vi "ZStepperPositionTest.vi"() -> ()   [LabVIEW 2014]
uses:
  inc/ThorZStepper.lvlib
panel:
  out "ZPosSlider":dbl(slide) caption="Z (mm)" min=-2.0 max=16.0 scale=-2.0..2.0
  in  "Z Stop":bool
  in  "Z Set Zero":bool
  in  "Tear Down Device and Stop Communication":bool
  out "status":i32
  in  "Move to New ZPos":bool
  in  "New ZPos (um)":dbl
  out "Current ZPos (mm)":dbl
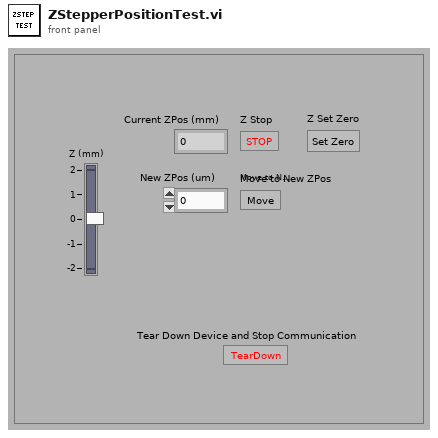
[diagram p1: front panel]
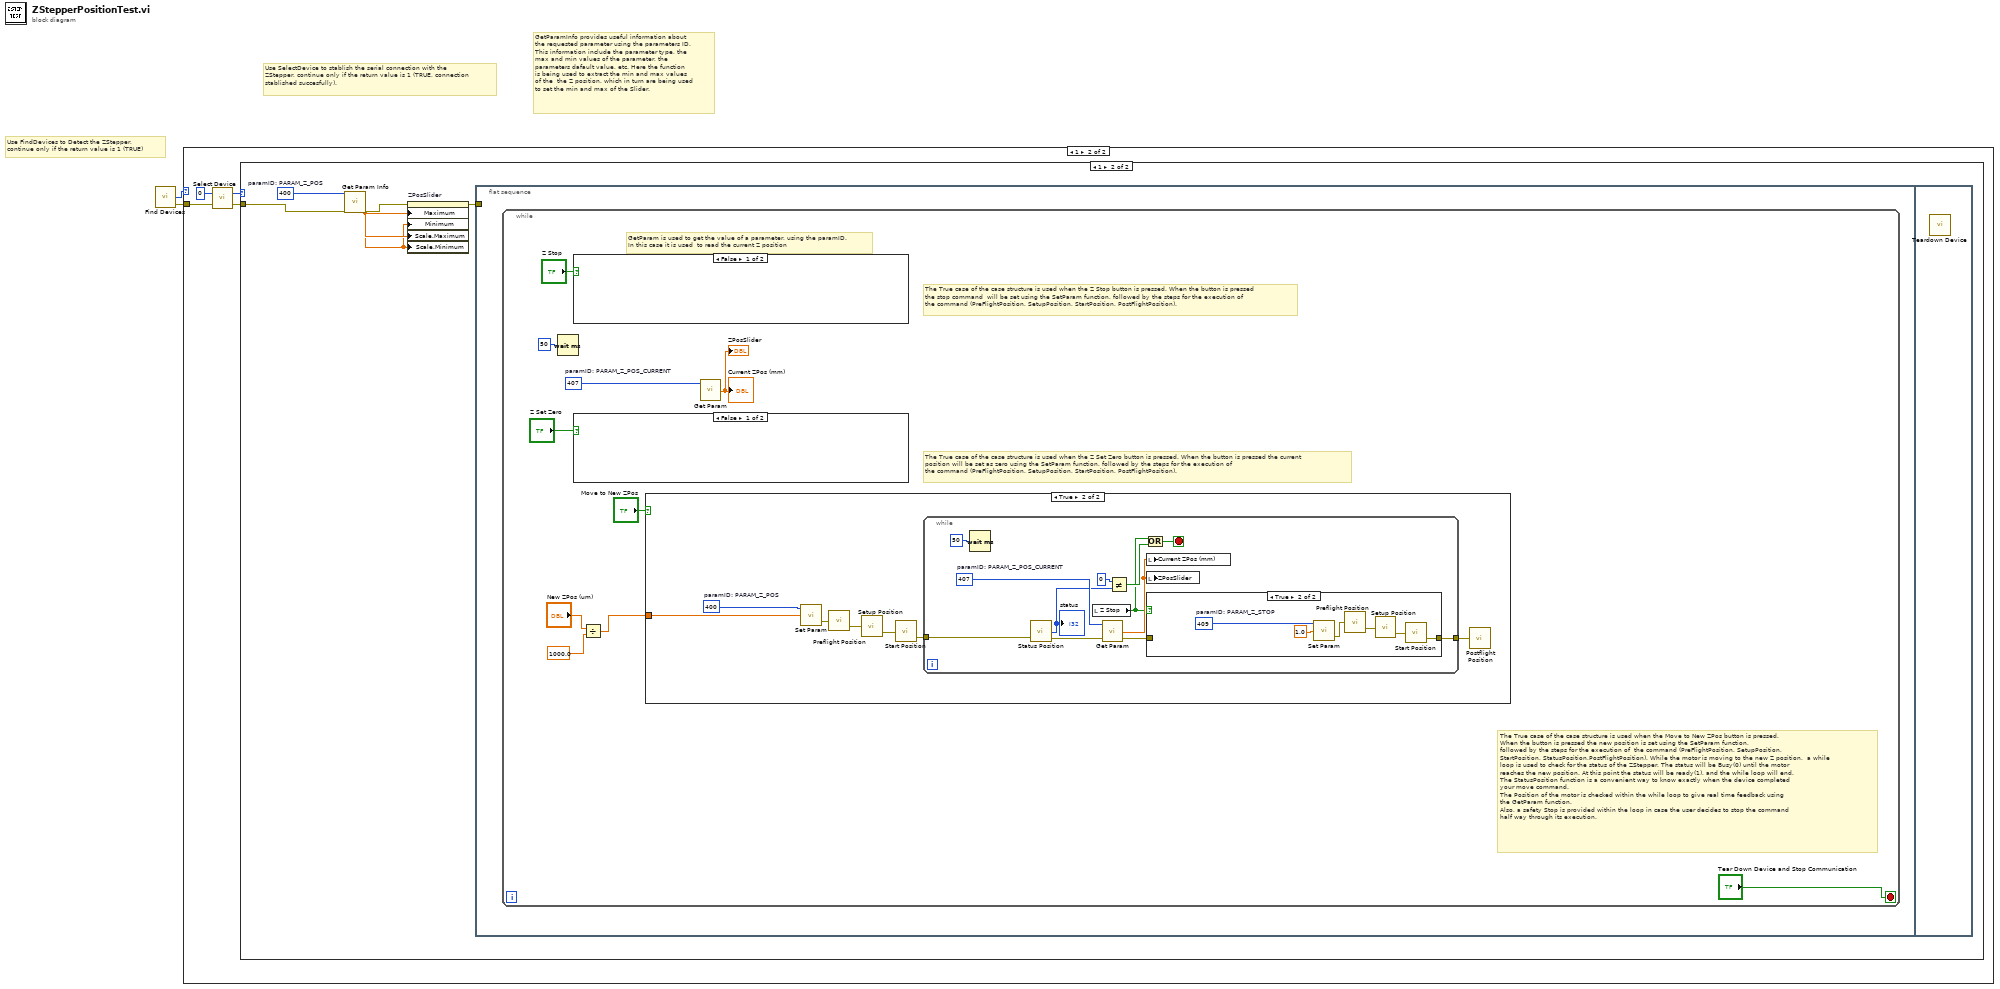
[diagram p0: block diagram]
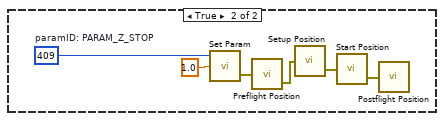
[diagram p4: hidden frame]
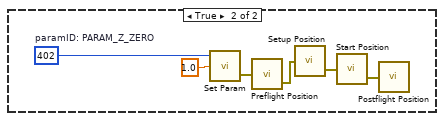
[diagram p5: hidden frame]
diagram:
  # "GetParamInfo provides useful information about \nthe requested parameter using the parameters ID.\nThis information include the parameter type, the \nmax and min values of the parameter, the \nparameters dafault value, etc. Here the function \nis being used to extract the min and max values \nof the  the Z position, which in turn are being used\nto set the min and max of the Slider."
  # "Use SelectDevice to stablish the serial connection with the\nZStepper, continue only if the return value is 1 (TRUE, connection\nstablished succesfully)."
  # "Use FindDevices to Detect the ZStepper, \ncontinue only if the return value is 1 (TRUE)"
  n1 = call "Find Devices.vi"() -> ("function return"=w1:i32, "error out"=w2:errorcluster)  [unwired: 2 in, 1 out]
  n2 = case shown="1" w1 {
    tunnel: w2 -> [_ w5]
    frame 0, Default {
    }
    frame 1 {
      n3 = call "Select Device.vi"("error in (no error)"=w5, "Device"=0) -> ("error out"=w3:errorcluster, "function return"=w4:i32)
      n4 = case shown="1" w4 {
        tunnel: w3 -> [_ w12]
        frame 0, Default {
        }
        frame 1 {
          w7 = 400  # paramID: PARAM_Z_POS
          n5 = call "Get Param Info.vi"("paramID"=w7, "error in (no error)"=w12) -> ("paramMin out"=w8:dbl, "paramMax out"=w9:dbl, "error out"=w10:errorcluster)  [unwired: 18 in, 5 out]
          n6 = property on="ZPosSlider" class="Slide (strict)"(error in=w10, "Maximum"=w9, "Minimum"=w8, "Scale.Maximum"=w9, "Scale.Minimum"=w8) -> (error out=w11:errorcluster)  [unwired: 1 in, 1 out]
          n7 = flat-sequence {
            tunnel: w11 -> [_]
            frame #0 {
              n8 = while {
                stop <- "Tear Down Device and Stop Communication" stop-if-true
                w20 = 407  # paramID: PARAM_Z_POS_CURRENT
                # "The True case of the case structure is used when the Move to New ZPos button is pressed. \nWhen the button is pressed the new position is set using the SetParam function, \nfollowed by the steps for the execution of  the command (PreFlightPosition, SetupPosition, \nStartPosition, StatusPosition,PostFlightPosition). While the motor is moving to the new Z position,  a while \nloop is used to check for the status of the ZStepper. The status will be Busy(0) until the motor\nreaches the new position. At this point the status will be ready(1), and the while loop will end.\nThe StatusPosition function is a convenient way to know exactly when the device completed\nyour move command.\nThe Position of the motor is checked within the while loop to give real time feedback using \nthe GetParam function.\nAlso, a safety Stop is provided within the loop in case the user decides to stop the command \nhalf way through its execution."
                # "The True case of the case structure is used when the Z Stop button is pressed. When the button is pressed\nthe stop command  will be set using the SetParam function, followed by the steps for the execution of \nthe command (PreFlightPosition, SetupPosition, StartPosition, PostFlightPosition)."
                # "GetParam is used to get the value of a parameter, using the paramID.\nIn this case it is used  to read the current Z position"
                # "The True case of the case structure is used when the Z Set Zero button is pressed. When the button is pressed the current\nposition will be set as zero using the SetParam function, followed by the steps for the execution of \nthe command (PreFlightPosition, SetupPosition, StartPosition, PostFlightPosition)."
                n9 = Wait (ms)(milliseconds to wait=u32 50) -> ()  [unwired: 1 out]
                n10 = case shown="False" "Z Stop" {
                  frame False {
                  }
                  frame True {
                    w27 = 409  # paramID: PARAM_Z_STOP
                    n11 = call "Set Param.vi"("param"=1.0, "paramID"=w27) -> ("error out"=w26:errorcluster)  [unwired: 1 in, 1 out]
                    n12 = call "Preflight Position.vi"("error in (no error)"=w26) -> ("error out"=w25:errorcluster)  [unwired: 1 out]
                    n13 = call "Setup Position.vi"("error in (no error)"=w25) -> ("error out"=w24:errorcluster)  [unwired: 1 out]
                    n14 = call "Start Position.vi"("error in (no error)"=w24) -> ("error out"=w23:errorcluster)  [unwired: 1 out]
                    n15 = call "Postflight Position.vi"("error in (no error)"=w23) -> ()  [unwired: 2 out]
                  }
                }
                n16 = case shown="False" "Z Set Zero" {
                  frame False {
                  }
                  frame True {
                    w33 = 402  # paramID: PARAM_Z_ZERO
                    n17 = call "Set Param.vi"("param"=1.0, "paramID"=w33) -> ("error out"=w32:errorcluster)  [unwired: 1 in, 1 out]
                    n18 = call "Preflight Position.vi"("error in (no error)"=w32) -> ("error out"=w31:errorcluster)  [unwired: 1 out]
                    n19 = call "Setup Position.vi"("error in (no error)"=w31) -> ("error out"=w30:errorcluster)  [unwired: 1 out]
                    n20 = call "Start Position.vi"("error in (no error)"=w30) -> ("error out"=w29:errorcluster)  [unwired: 1 out]
                    n21 = call "Postflight Position.vi"("error in (no error)"=w29) -> ()  [unwired: 2 out]
                  }
                }
                n22 = Divide(x="New ZPos (um)", y=1000.0) -> (x/y=w14:dbl)
                n23 = case shown="True" "Move to New ZPos" {
                  tunnel: w14 -> [_ w37]
                  frame False {
                  }
                  frame True {
                    w39 = 400  # paramID: PARAM_Z_POS
                    n24 = call "Set Param.vi"("param"=w37, "paramID"=w39) -> ("error out"=w38:errorcluster)  [unwired: 1 in, 1 out]
                    n25 = call "Preflight Position.vi"("error in (no error)"=w38) -> ("error out"=w41:errorcluster)  [unwired: 1 out]
                    n26 = call "Setup Position.vi"("error in (no error)"=w41) -> ("error out"=w40:errorcluster)  [unwired: 1 out]
                    n27 = call "Start Position.vi"("error in (no error)"=w40) -> ("error out"=w36:errorcluster)  [unwired: 1 out]
                    n28 = while {
                      tunnel: w36 -> [w49]
                      tunnel: [w47] -> w35
                      stop <- w43 stop-if-true
                      w50 = 407  # paramID: PARAM_Z_POS_CURRENT
                      n29 = Wait (ms)(milliseconds to wait=u32 50) -> ()  [unwired: 1 out]
                      n30 = call "Status Position.vi"("error in (no error)"=w49) -> ("function return"=w45:i32, "error out"=w51:errorcluster)  [unwired: 1 in, 1 out]
                      "status" <- w45
                      n31 = local read "Z Stop"() -> (w42:bool)
                      n32 = call "Get Param.vi"("error in (no error)"=w51, "paramID"=w50) -> ("error out"=w48:errorcluster, "param out"=w46:dbl)  [unwired: 1 in, 1 out]
                      n33 = Not Equal?(x=0, y=w45) -> (x != y?=w44:bool)
                      n34 = Or(x=w42, y=w44) -> (x .or. y?=w43:bool)
                      n35 = local write "Current ZPos (mm)"(w46) -> ()
                      n36 = local write "ZPosSlider"(w46) -> ()
                      n37 = case shown="True" w42 {
                        tunnel: w48 -> [w54 _]
                        tunnel: [w54 w55] -> w47
                        frame False {
                        }
                        frame True {
                          w59 = 409  # paramID: PARAM_Z_STOP
                          n38 = call "Set Param.vi"("param"=1.0, "paramID"=w59) -> ("error out"=w58:errorcluster)  [unwired: 1 in, 1 out]
                          n39 = call "Preflight Position.vi"("error in (no error)"=w58) -> ("error out"=w57:errorcluster)  [unwired: 1 out]
                          n40 = call "Setup Position.vi"("error in (no error)"=w57) -> ("error out"=w56:errorcluster)  [unwired: 1 out]
                          n41 = call "Start Position.vi"("error in (no error)"=w56) -> ("error out"=w55:errorcluster)  [unwired: 1 out]
                        }
                      }
                    }
                    n42 = call "Postflight Position.vi"("error in (no error)"=w35) -> ()  [unwired: 2 out]
                  }
                }
                n43 = call "Get Param.vi"("paramID"=w20) -> ("param out"=→"Current ZPos (mm)" →"ZPosSlider":dbl)  [unwired: 2 in, 2 out]
              }
            }
            frame #1 {
              n44 = call "Teardown Device.vi"() -> ()  [unwired: 1 in, 2 out]
            }
          }
        }
      }
    }
  }
